vi "createSimpleArray.vi"(1 "nbpoint1":dbl, 2 "Bgstop":dbl, 3 "Bgstart":dbl) -> (0 "Outarray":dbl[](array[numeric]))   [LabVIEW 2011]
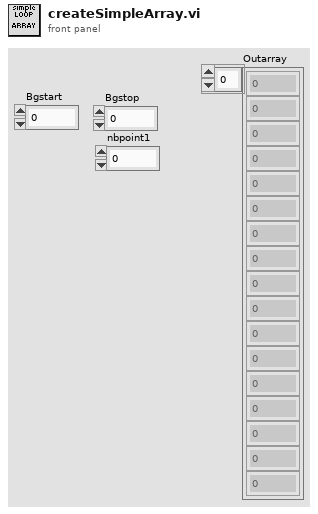
[diagram p1: front panel]
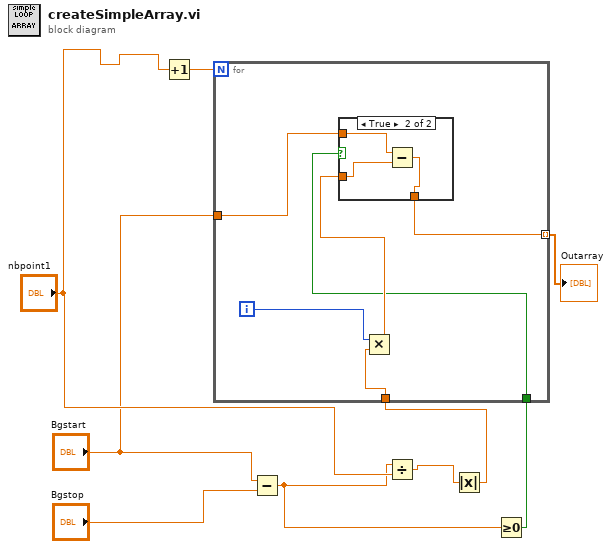
[diagram p0: block diagram]
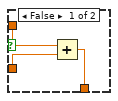
[diagram p2: hidden frame]
diagram:
  n1 = Increment(x="nbpoint1") -> (x+1=w9:dbl)
  n2 = Subtract(x="Bgstart", y="Bgstop") -> (x-y=w2:dbl)
  n3 = Divide(x=w2, y="nbpoint1") -> (x/y=w6:dbl)
  n4 = Absolute Value(x=w6) -> (abs(x)=w5:dbl)
  n5 = Greater Or Equal To 0?(x=w2) -> (x >= 0?=w1:bool)
  n6 = for {
    N: w9 -> [_]
    tunnel: w5 -> [w14]
    tunnel: "Bgstart" -> [w13]
    tunnel: [w11] -> w3 mode=indexing
    tunnel: w1 -> [w10]
    i -> [w15]
    n7 = Multiply(x=w15, y=w14) -> (x*y=w12:dbl)
    n8 = case shown="True" w10 {
      tunnel: w13 -> [w18 w21]
      tunnel: w12 -> [w17 w20]
      tunnel: [w16 w19] -> w11
      frame False {
        n9 = Add(x=w18, y=w17) -> (x+y=w16:dbl)
      }
      frame True {
        n10 = Subtract(x=w21, y=w20) -> (x-y=w19:dbl)
      }
    }
  }
  "Outarray" <- w3
